vi "8.8.3_기능적 글로벌.vi"(2 "입력":dbl, 3 "명령":enum16{"값 쓰기", "값 읽기"}(ring)) -> (0 "출력":dbl)   [LabVIEW 2018]
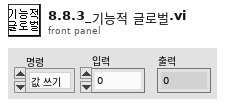
[diagram p1: front panel]
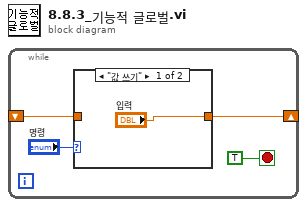
[diagram p0: block diagram]
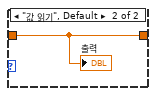
[diagram p2: hidden frame]
diagram:
  n1 = while {
    shift-right: [w1] -> _
    shift-left: _ -> [w2]
    stop <- TRUE stop-if-true
    n2 = case shown="\"값 쓰기\"" "명령" {
      tunnel: w2 -> [_ w6]
      tunnel: ["입력" w6] -> w1
      frame "값 쓰기" {
      }
      frame "값 읽기", Default {
        "출력" <- w6
      }
    }
  }
